vi "BL132 CAM4end.vi"() -> ()   [LabVIEW 2015]
panel:
  out "APX PREP SIDE":T1(plugin-control)
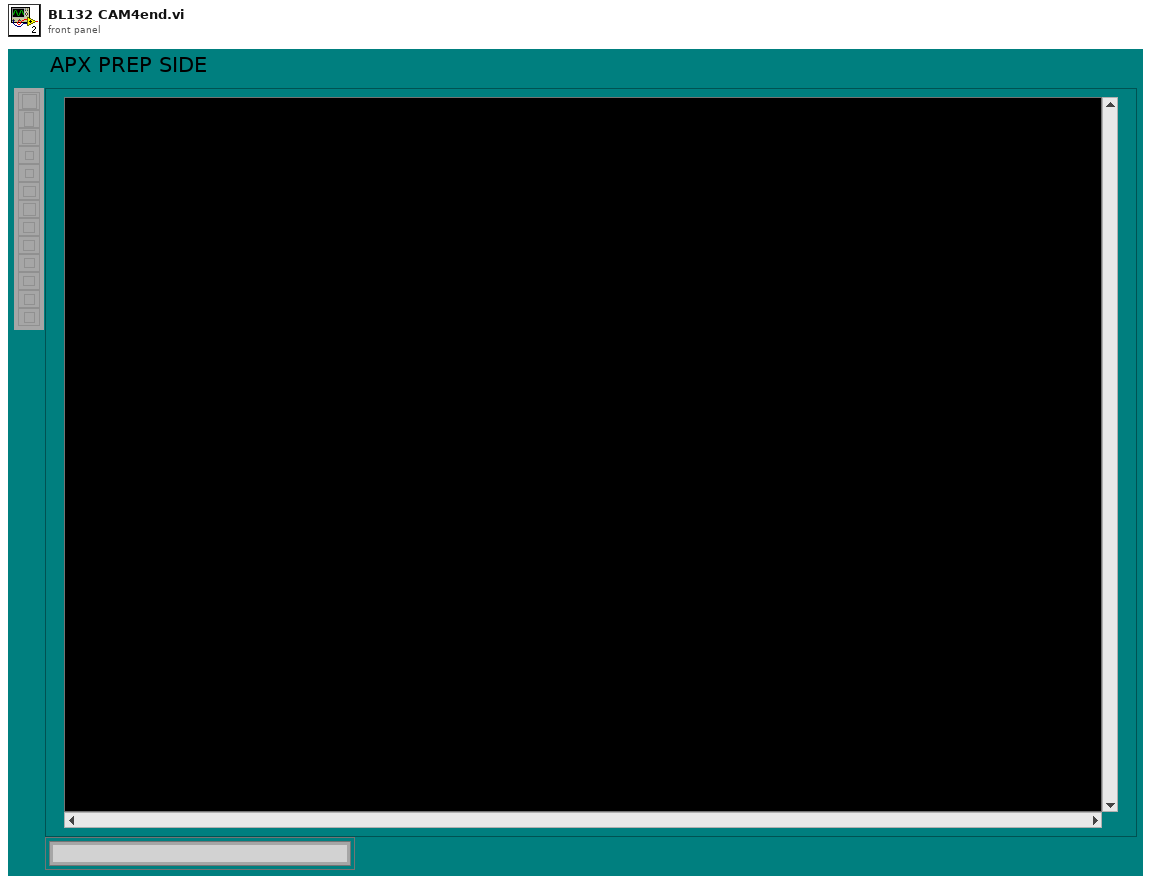
[diagram p1: front panel]
types:
  T1 = typedef "IMAQ Image.ctl" = refnum<image>
  T2 = cluster{"Pattern":i32, "Algorithm":i32, "Red Gain":dbl, "Green Gain":dbl, "Blue Gain":dbl}
  T3 = typedef "Image Type" = u32
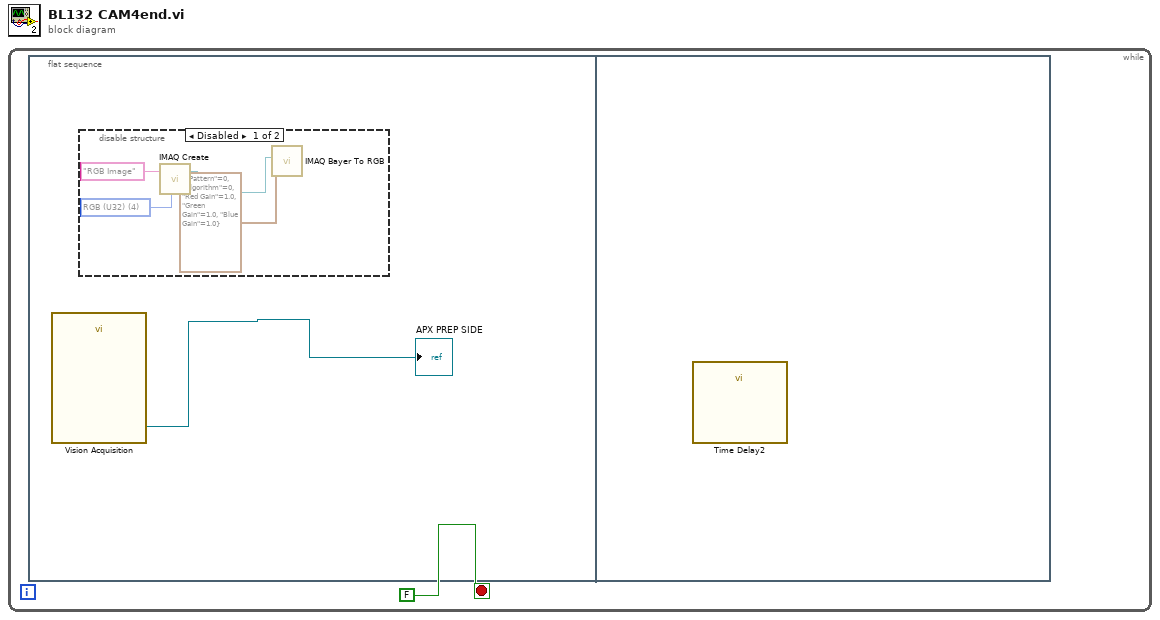
[diagram p0: block diagram]
diagram:
  n1 = while {
    stop <- FALSE stop-if-true
    n2 = flat-sequence {
      frame #0 {
        n3 = call "Vision Acquisition"() -> ("Image Out"=→"APX PREP SIDE":T1)  [unwired: 26 in, 1 out]
        n4 = disable-structure shown="Disabled" {
          frame Disabled {
            w4 = T3 4 items=["Grayscale (U8)", "Grayscale (I16)", "Grayscale (SGL)", "Complex (CSG)", "RGB (U32)", "HSL (U32)", "RGB (U64)", "Grayscale (U16)"] ("Image Type")
            n5 = call "IMAQ Create"("Image Name"="RGB Image", "Image Type"=w4) -> ("New Image"=w3:T1)  [unwired: 2 in, 2 out]
            n6 = call "IMAQ Bayer To RGB"("Bayer Parameters"=T2 {"Pattern"=0, "Algorithm"=0, "Red Gain"=1.0, "Green Gain"=1.0, "Blue Gain"=1.0}, "Image Dst"=w3) -> ()  [unwired: 8 in, 2 out]
          }
          frame Enabled {
          }
        }
      }
      frame #1 {
        n7 = call "Time Delay2"() -> ()  [unwired: 11 in, 1 out]
      }
    }
  }
